vi "RichToFlatni_xnet_can_bm_api_ErrorInfo.vi"(5 "OutputClusterType":T1, 11 "InputCluster":T2) -> (3 "OutputCluster":T1)   [LabVIEW 2025, in "xnet_can_bus_monitor_api_client.lvlib"]
uses:
  ni_xnet_can_bm_api_ErrorInfo.ctl
  ni_xnet_can_bm_api_ErrorInfo_Flat.ctl
  xnet_can_bus_monitor_api_client.lvlib
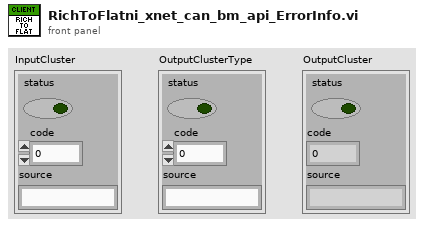
[diagram p1: front panel]
types:
  T1 = typedef "xnet_can_bus_monitor_api_client.lvlib/ni_xnet_can_bm_api_ErrorInfo_Flat.ctl" = errorcluster
  T2 = typedef "xnet_can_bus_monitor_api_client.lvlib/ni_xnet_can_bm_api_ErrorInfo.ctl" = errorcluster
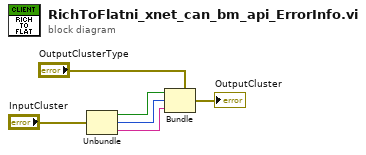
[diagram p0: block diagram]
diagram:
  n1 = Unbundle "Unbundle"("InputCluster") -> ("status"=w3:bool, "code"=w2:i32, "source"=w1:string)
  n2 = Bundle "Bundle"(cluster="OutputClusterType", "status"=w3, "code"=w2, "source"=w1) -> (→"OutputCluster":T1)
